vi "Data logger Array Enqueue Function.vi"(0 "QRef in":refnum<queue>, 5 "Array of Messages":T1[](array[typedef]), 11 "Error in":errorcluster, 13 "Mode":enum16{"Back", "Front", "Replace"}(ring)) -> (4 "QRef out":refnum<queue>, 15 "Error out":errorcluster)   [LabVIEW 2014]
uses:
  TypeDef/Q1 Message.ctl
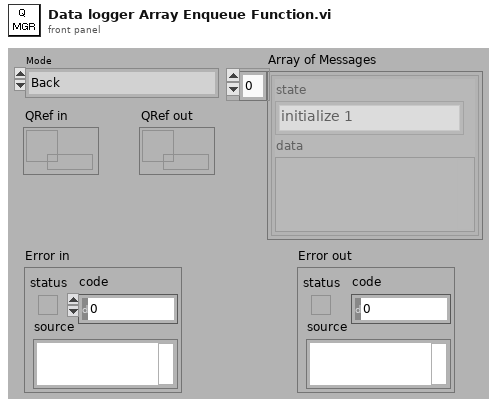
[diagram p1: front panel]
types:
  T1 = typedef "Q1 Message.ctl" = cluster{"state":enum16{"initialize 1", "initialize 2", "initialize 3", "initialize 4", "initialize 5", "initialize 6", "initialize 7", "initialize 8", "initialize 9", "Idle", "Preparation 1", "Preparation 2", "Preparation 3", "Preparation 4", "Record", "Stop recording", "Exit", "Defrag", "View", "Create Database", "Update folder setting", "Update Preference", "Update TDMS properties", "CSV Delimiter", "DB Type", "Hidden Processes", "Replace Database", "Logged File Viewer", "Defrag Prompt File", "View Prompt File", "Save to config file", "Open from config file"}, "data":variant}
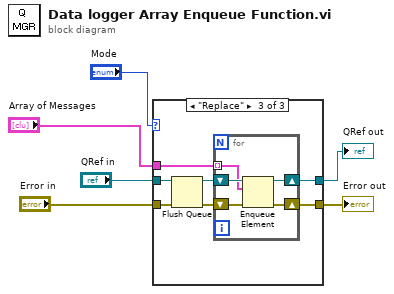
[diagram p0: block diagram]
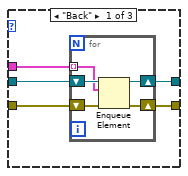
[diagram p2: hidden frame]
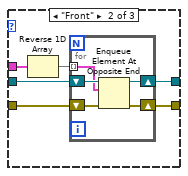
[diagram p3: hidden frame]
diagram:
  n1 = case shown="\"Replace\"" "Mode" {
    tunnel: "Array of Messages" -> [w9 w22 w32]
    tunnel: "QRef in" -> [w11 w20 w34]
    tunnel: [w10 w19 w31] -> w2
    tunnel: "Error in" -> [w8 w18 w29]
    tunnel: [w7 w17 w28] -> w6
    frame "Back" {
      n2 = for {
        shift-right: [w15] -> w10
        shift-left: w11 -> [w16]
        tunnel: w9 -> [w14] mode=indexing
        shift-right: [w12] -> w7
        shift-left: w8 -> [w13]
        n3 = Enqueue Element(queue=w16, element=w14, error in (no error)=w13) -> (queue out=w15:refnum<queue>, error out=w12:errorcluster)  [unwired: 1 in, 1 out]
      }
    }
    frame "Front" {
      n4 = Reverse 1D Array(array=w22) -> (reversed array=w21:T1[])
      n5 = for {
        tunnel: w21 -> [w26] mode=indexing
        shift-right: [w25] -> w19
        shift-left: w20 -> [w27]
        shift-right: [w23] -> w17
        shift-left: w18 -> [w24]
        n6 = Enqueue Element At Opposite End(queue=w27, element=w26, error in (no error)=w24) -> (queue out=w25:refnum<queue>, error out=w23:errorcluster)  [unwired: 1 in, 1 out]
      }
    }
    frame "Replace" {
      n7 = Flush Queue(queue=w34, error in (no error)=w29) -> (queue out=w33:refnum<queue>, error out=w30:errorcluster)  [unwired: 1 out]
      n8 = for {
        tunnel: w32 -> [w38] mode=indexing
        shift-right: [w37] -> w31
        shift-left: w33 -> [w39]
        shift-right: [w35] -> w28
        shift-left: w30 -> [w36]
        n9 = Enqueue Element(queue=w39, element=w38, error in (no error)=w36) -> (queue out=w37:refnum<queue>, error out=w35:errorcluster)  [unwired: 1 in, 1 out]
      }
    }
  }
  "Error out" <- w6
  "QRef out" <- w2
